vi "application options.vi"() -> (2 "help message":string, 3 "Options":T1[](array[typedef]))   [LabVIEW 2024]
uses:
  <vilib>/Wiresmith Technology/G CLI/Argument Parser/Option Class/Option Configuration.ctl
  <vilib>/Wiresmith Technology/G CLI/Argument Parser/Option Class/Argument Type.ctl
  <vilib>/Wiresmith Technology/G CLI/Argument Parser/Option Class/Option.lvclass
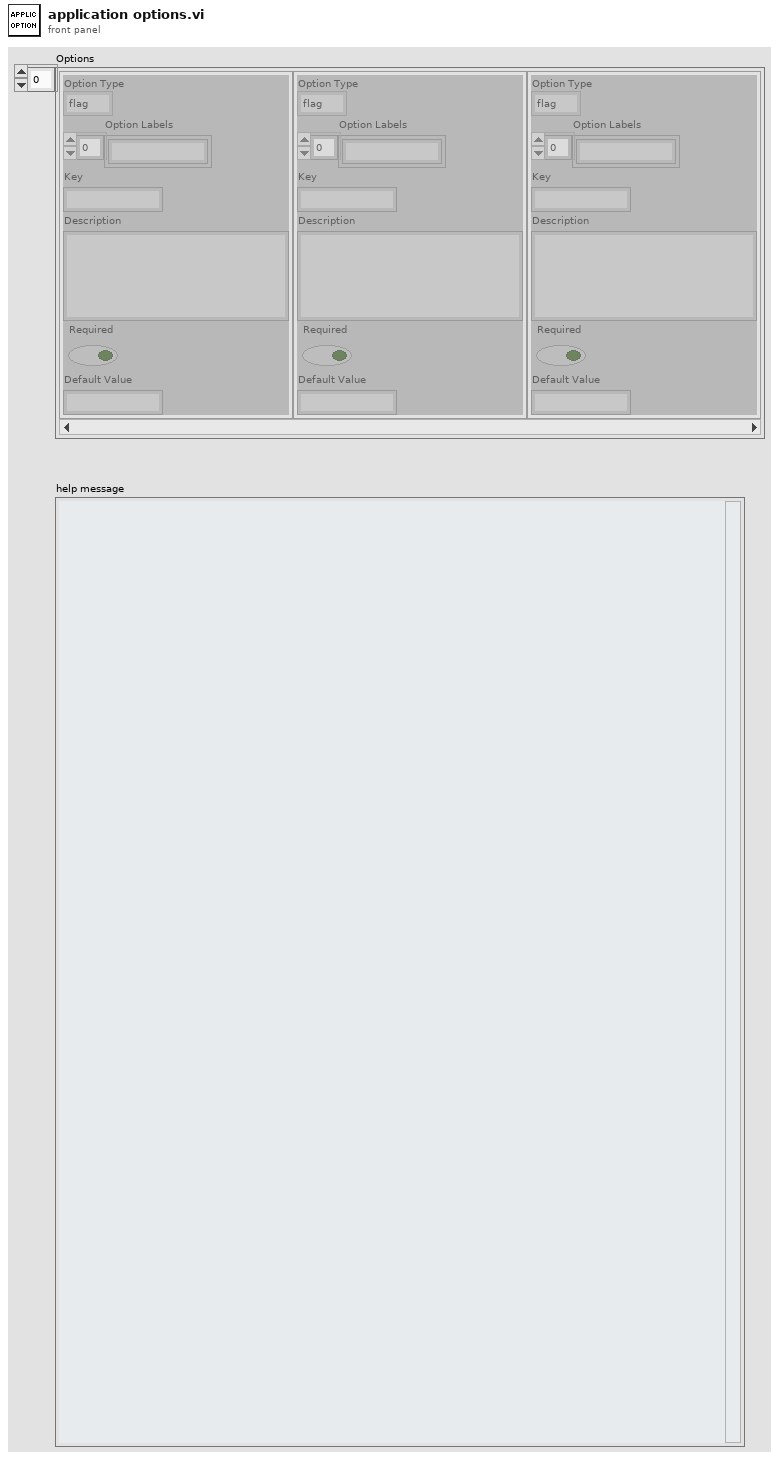
[diagram p1: front panel]
types:
  T1 = typedef "Option Parser.lvlib/Option.lvclass/Option Configuration.ctl" = cluster{"Option Type":T2, "Option Labels":string[], "Key":string, "Description":string, "Required":bool, "Default Value":string}
  T2 = typedef "Option Parser.lvlib/Option.lvclass/Argument Type.ctl" = enum16{"flag", "value"}
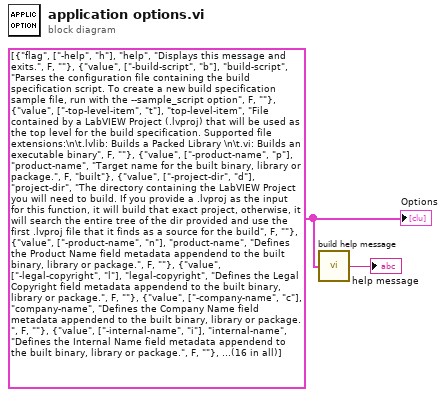
[diagram p0: block diagram]
diagram:
  w2 = T1[] [{"Option Type"=enum."flag", "Option Labels"=["-help", "h"], "Key"="help", "Description"="Displays this message and exits.", "Required"=FALSE, "Default Value"=""}, {"Option Type"=enum."value", "Option Labels"=["-build-script", "b"], "Key"="build-script", "Description"="Parses the configuration file containing the build specification script. To create a new build specification sample file, run with the --sample_script option", "Required"=FALSE, "Default Value"=""}, {"Option Type"=enum."value", "Option Labels"=["-top-level-item", "t"], "Key"="top-level-item", "Description"="File contained by a LabVIEW Project (.lvproj) that will be used as the top level for the build specification. Supported file extensions:\n\t.lvlib: Builds a Packed Library \n\t.vi: Builds an executable binary", "Required"=FALSE, "Default Value"=""}, {"Option Type"=enum."value", "Option Labels"=["-product-name", "p"], "Key"="product-name", "Description"="Target name for the built binary, library or package.", "Required"=FALSE, "Default Value"="built"}, {"Option Type"=enum."value", "Option Labels"=["-project-dir", "d"], "Key"="project-dir", "Description"="The directory containing the LabVIEW Project you will need to build. If you provide a .lvproj as the input for this function, it will build that exact project, otherwise, it will search the entire tree of the dir provided and use the first .lvproj file that it finds as a source for the build", "Required"=FALSE, "Default Value"=""}, {"Option Type"=enum."value", "Option Labels"=["-product-name", "n"], "Key"="product-name", "Description"="Defines the Product Name field metadata appendend to the built binary, library or package.", "Required"=FALSE, "Default Value"=""}, {"Option Type"=enum."value", "Option Labels"=["-legal-copyright", "l"], "Key"="legal-copyright", "Description"="Defines the Legal Copyright field metadata appendend to the built binary, library or package.", "Required"=FALSE, "Default Value"=""}, {"Option Type"=enum."value", "Option Labels"=["-company-name", "c"], "Key"="company-name", "Description"="Defines the Company Name field metadata appendend to the built binary, library or package.", "Required"=FALSE, "Default Value"=""}, {"Option Type"=enum."value", "Option Labels"=["-internal-name", "i"], "Key"="internal-name", "Description"="Defines the Internal Name field metadata appendend to the built binary, library or package.", "Required"=FALSE, "Default Value"=""}, {"Option Type"=enum."value", "Option Labels"=["-file-description", "F"], "Key"="file-description", "Description"="Defines the File Description field metadata appendend to the built binary, library or package.", "Required"=FALSE, "Default Value"=""}, {"Option Type"=enum."value", "Option Labels"=["-pre-build-vi", "B"], "Key"="pre-build-vi", "Description"="File path of the pre-build vi that will be executed before the build takes place.", "Required"=FALSE, "Default Value"=""}, {"Option Type"=enum."value", "Option Labels"=["-post-build-vi", "b"], "Key"="post-build-vi", "Description"="File path of the post-build vi that will be executed after a successful build finishes.", "Required"=FALSE, "Default Value"=""}, {"Option Type"=enum."value", "Option Labels"=["-files-to-include", "I"], "Key"="files-to-include", "Description"="List of files to include in the target build directory. Formatted with Windows-type slashes for directories (backward slashes).\n\nAccepts either a relative path defined in relation to the .lvproj used for the build, or a list of absolute paths to the desired items.\n\nExample: \n\n.\\file1.jpg .\\docs\\doc1.html C:\\folder\\file2.txt", "Required"=FALSE, "Default Value"=""}, {"Option Type"=enum."value", "Option Labels"=["-version-major", "M"], "Key"="version-major", "Description"="Updates the binary, package or library with the specified Major version in Semantic Versioning standard.", "Required"=FALSE, "Default Value"=""}, {"Option Type"=enum."value", "Option Labels"=["-version-minor", "m"], "Key"="version-minor", "Description"="Updates the binary, package or library with the specified Minor version in Semantic Versioning standard.", "Required"=FALSE, "Default Value"=""}, {"Option Type"=enum."value", "Option Labels"=["-version-bugfix", "g"], "Key"="version-bugfix", "Description"="Updates the binary, package or library with the specified Bugfix version in Semantic Versioning standard.", "Required"=FALSE, "Default Value"=""}] ("Options")
  n1 = call "build help message.vi"("Options"=w2) -> ("help"=→"help message":string)
  "Options" <- w2
